vi "set_subpattern.vi"(6 "diameter":dbl, 7 "height":dbl, 8 "error in (no error)":errorcluster, 9 "number of iteration points":dbl, 10 "winding number":dbl, 11 "TrajectoryMH100122AODRAPS in":refnum<class "TrajectoryMH100122AODRAPS.lvclass">) -> (0 "error out":errorcluster, 3 "TrajectoryMH100122AODRAPS out":refnum<class "TrajectoryMH100122AODRAPS.lvclass">)   [LabVIEW 2010, in "TrajectoryMH100122AODRAPS.lvclass"]
uses:
  TrajectoryMH100122AODRAPS.lvclass
  TrajectoryMH100122AODRAPS.lvclass/TrajectoryMH100122AODRAPS.ctl
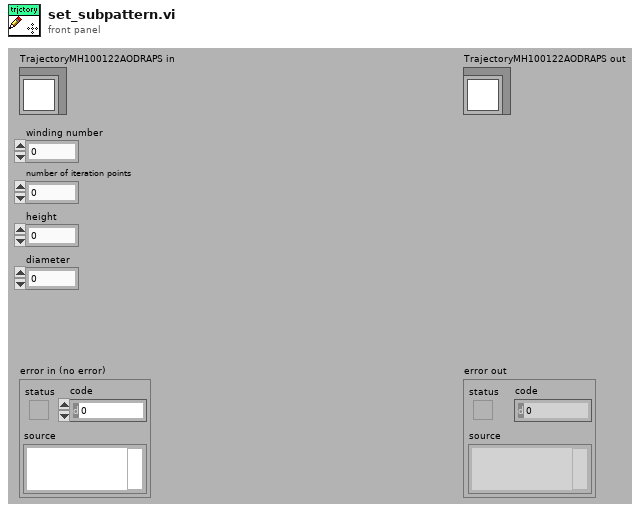
[diagram p1: front panel]
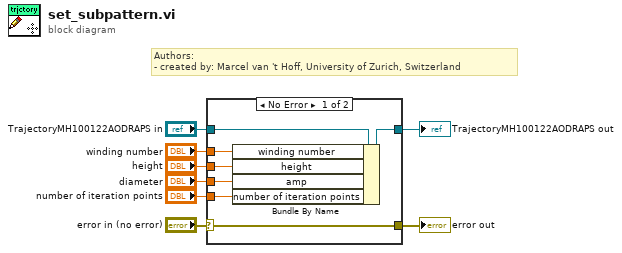
[diagram p0: block diagram]
diagram:
  # "Authors: \n- created by: Marcel van 't Hoff, University of Zurich, Switzerland"
  n1 = case shown="No Error" "error in (no error)" {
    selector: "error in (no error)" -> [w15 w17]
    tunnel: [w15 w17] -> w7
    tunnel: [w13 w16] -> w5
    tunnel: "TrajectoryMH100122AODRAPS in" -> [w14 w16]
    tunnel: "winding number" -> [w12 _]
    tunnel: "height" -> [w11 _]
    tunnel: "diameter" -> [w10 _]
    tunnel: "number of iteration points" -> [w9 _]
    frame No Error {
      n2 = Bundle By Name(cluster=w14, "winding number"=w12, "height"=w11, "amp"=w10, "number of iteration points"=w9) -> (w13:refnum<class "TrajectoryMH100122AODRAPS.lvclass">)
    }
    frame Error {
    }
  }
  "error out" <- w7
  "TrajectoryMH100122AODRAPS out" <- w5
